vi "UpdateErrorCode.vi"(8 "error in (no error)":errorcluster, 9 "Error":bool, 10 "ErrorBit":u8, 11 "MFActor in":refnum<class "MFActor.lvclass">) -> (0 "error out":errorcluster, 3 "MFActor out":refnum<class "MFActor.lvclass">)   [LabVIEW 2024, in "MFActor.lvlib" / "MFActor.lvclass"]
uses:
  MFActor.lvclass
  MFActor.lvclass/MFActor.ctl
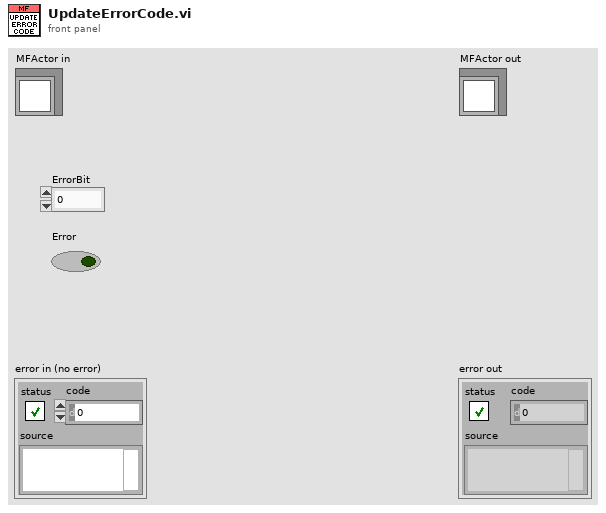
[diagram p1: front panel]
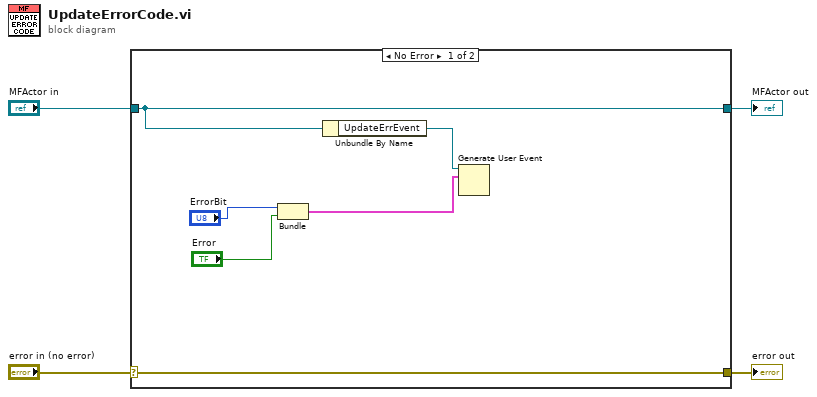
[diagram p0: block diagram]
diagram:
  n1 = case shown="No Error" "error in (no error)" {
    selector: "error in (no error)" -> [w10 w12]
    tunnel: [w10 w12] -> w3
    tunnel: [w5 w11] -> w1
    tunnel: "MFActor in" -> [w5 w11]
    frame No Error {
      n2 = Bundle("ErrorBit"="ErrorBit", "Error"="Error") -> (w6:cluster{"ErrorBit":u8, "Error":bool})  [unwired: 1 in]
      n3 = Unbundle By Name(w5) -> ("UpdateErrEvent"=w9:refnum<user-event>)
      n4 = Generate User Event(user event=w9, event data cluster=w6) -> ()  [unwired: 2 in, 2 out]
    }
    frame Error {
    }
  }
  "error out" <- w3
  "MFActor out" <- w1
